vi "Read Output.vi"(8 "error in (no error)":errorcluster, 10 "Channel (1)":string="1", 11 "VISA resource name":refnum<visa-resource-name>) -> (0 "error out":errorcluster, 1 "Actual Current Level (A)":dbl[](array[numeric]) format="%.2g", 2 "Actual Voltage Level (V)":dbl[](array[numeric]) format="%.2g", 3 "VISA resource name out":refnum<visa-resource-name>)   [LabVIEW 2020, in "Keysight E36300 Series.lvlib"]
doc: "Returns the actual voltage level and actual current level for a desired channel."
uses:
  Keysight E36300 Series.lvlib
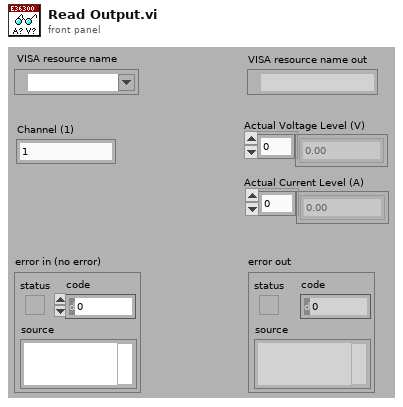
[diagram p1: front panel]
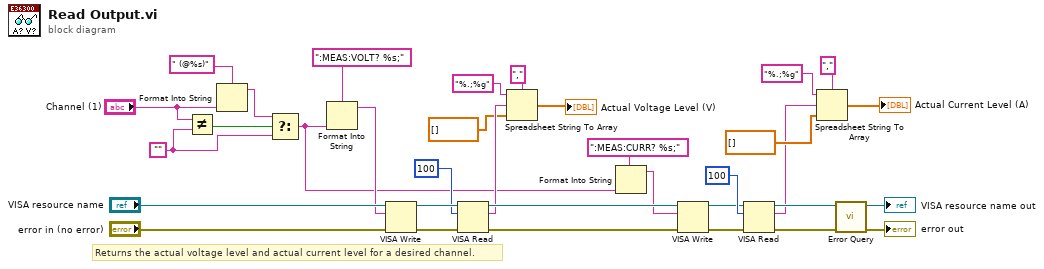
[diagram p0: block diagram]
diagram:
  w1 = ""
  # "Returns the actual voltage level and actual current level for a desired channel."
  n1 = Not Equal?(x="Channel (1)", y=w1) -> (x != y?=w4:bool)
  n2 = Format Into String(format string=" (@%s)", "Channel (1)") -> (resulting string=w5:string)  [unwired: 2 in, 1 out]
  n3 = Select(t=w5, s=w4, f=w1) -> (s? t:f=w2:string)
  n4 = Format Into String(format string=":MEAS:VOLT? %s;", w2) -> (resulting string=w19:string)  [unwired: 2 in, 1 out]
  n5 = VISA Write(VISA resource name="VISA resource name", write buffer=w19, error in (no error)="error in (no error)") -> (VISA resource name out=w33:refnum<visa-resource-name>, error out=w34:errorcluster)  [unwired: 1 out]
  n6 = VISA Read(VISA resource name=w33, byte count=u32 100, error in (no error)=w34) -> (VISA resource name out=w23:refnum<visa-resource-name>, read buffer=w14:string, error out=w24:errorcluster)  [unwired: 1 out]
  n7 = Spreadsheet String To Array(delimiter (Tab)=",", format string="%.;%g", spreadsheet string=w14, array type (2D Dbl)=dbl[] []) -> (array=→"Actual Voltage Level (V)":dbl[])
  n8 = Format Into String(format string=":MEAS:CURR? %s;", w2) -> (resulting string=w17:string)  [unwired: 2 in, 1 out]
  n9 = VISA Write(VISA resource name=w23, write buffer=w17, error in (no error)=w24) -> (VISA resource name out=w28:refnum<visa-resource-name>, error out=w27:errorcluster)  [unwired: 1 out]
  n10 = VISA Read(VISA resource name=w28, byte count=u32 100, error in (no error)=w27) -> (VISA resource name out=w26:refnum<visa-resource-name>, read buffer=w9:string, error out=w25:errorcluster)  [unwired: 1 out]
  n11 = Spreadsheet String To Array(delimiter (Tab)=",", format string="%.;%g", spreadsheet string=w9, array type (2D Dbl)=dbl[] []) -> (array=→"Actual Current Level (A)":dbl[])
  n12 = call "Error Query.vi"("error in (no error)"=w25, "VISA resource name"=w26) -> ("error out"=→"error out":errorcluster, "VISA resource name out"=→"VISA resource name out":refnum<visa-resource-name>)  [unwired: 6 in, 2 out]
